vi "GetClampResultNames.vi"(7 "ProjectName":string="Prj", 10 "data":T2={"Clamp Settings"={"Contrast"=40, "Filter width"=4, "Steepness"=2, "Subsampling Ratio"=5, "Show Search Area"=TRUE, "Show Search Lines"=TRUE, "Show Edges Found"=TRUE, "Show Result"=TRUE}, "ROI Descriptor"={"Global Rectangle"=[], "Contours"=[]}, "Process"=0}, 11 "ROI_Name":string="ROI1") -> (3 "ResultNames":string[](array[string]))   [LabVIEW 2019]
uses:
  Controls/Clamp/Analysis_Clamp_Parameter.ctl
  Controls/Clamp/Analysis_Clamp_Result.ctl
panel:
  in  "Analysis_Clamp_Result":T1 {"Edge Point"."Y" format="%.2f"; "Edge Point"."X" format="%.2f"}
  out "error out":errorcluster
  in  "error in (no error)":errorcluster
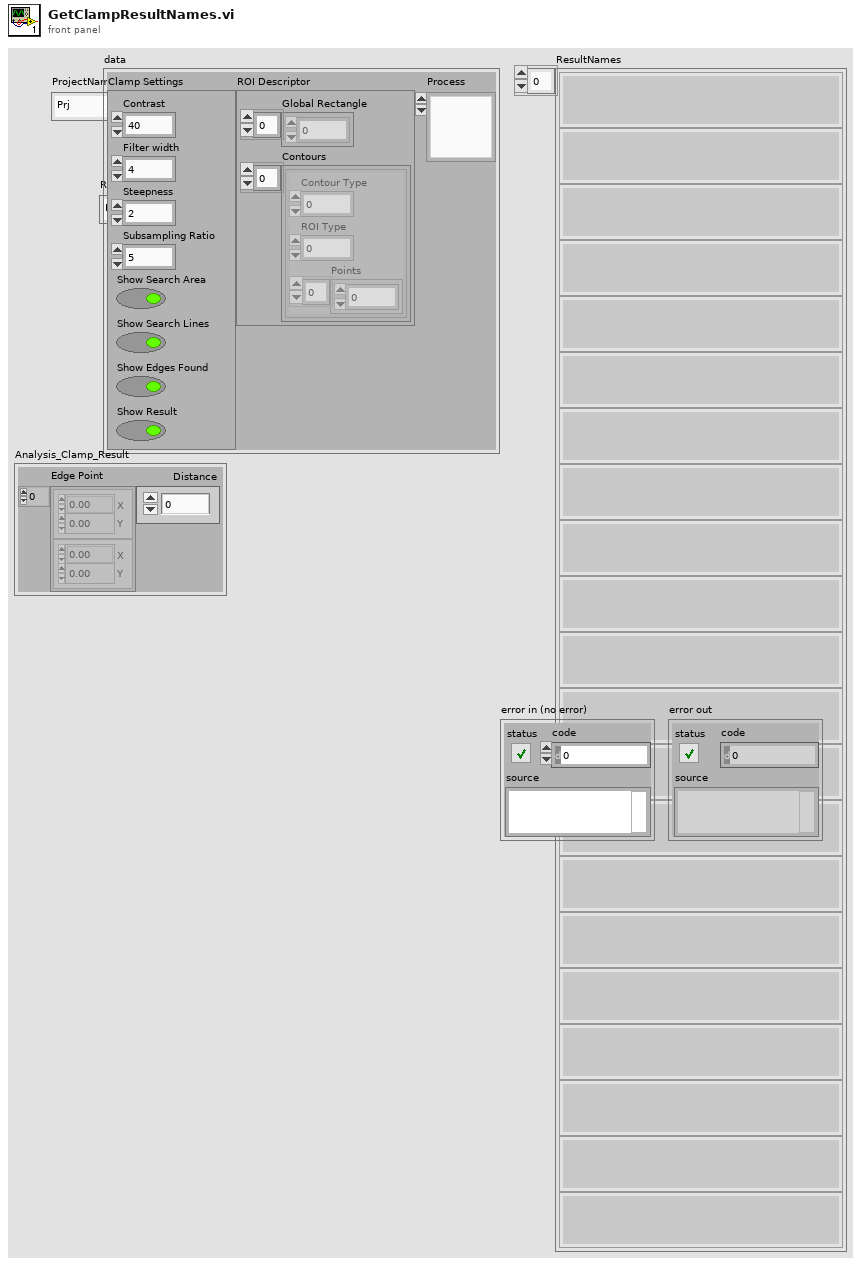
[diagram p1: front panel]
types:
  T1 = typedef "Analysis_Clamp_Result.ctl" = cluster{"Edge Point":cluster{"X":sgl, "Y":sgl}[], "Distance":sgl}
  T2 = typedef "Analysis_Clamp_Parameter.ctl" = cluster{"Clamp Settings":cluster{"Contrast":i32, "Filter width":i32, "Steepness":i32, "Subsampling Ratio":u32, "Show Search Area":bool, "Show Search Lines":bool, "Show Edges Found":bool, "Show Result":bool}, "ROI Descriptor":cluster{"Global Rectangle":i32[], "Contours":cluster{"Contour Type":u32, "ROI Type":u32, "Points":i32[]}[]}, "Process":u16}
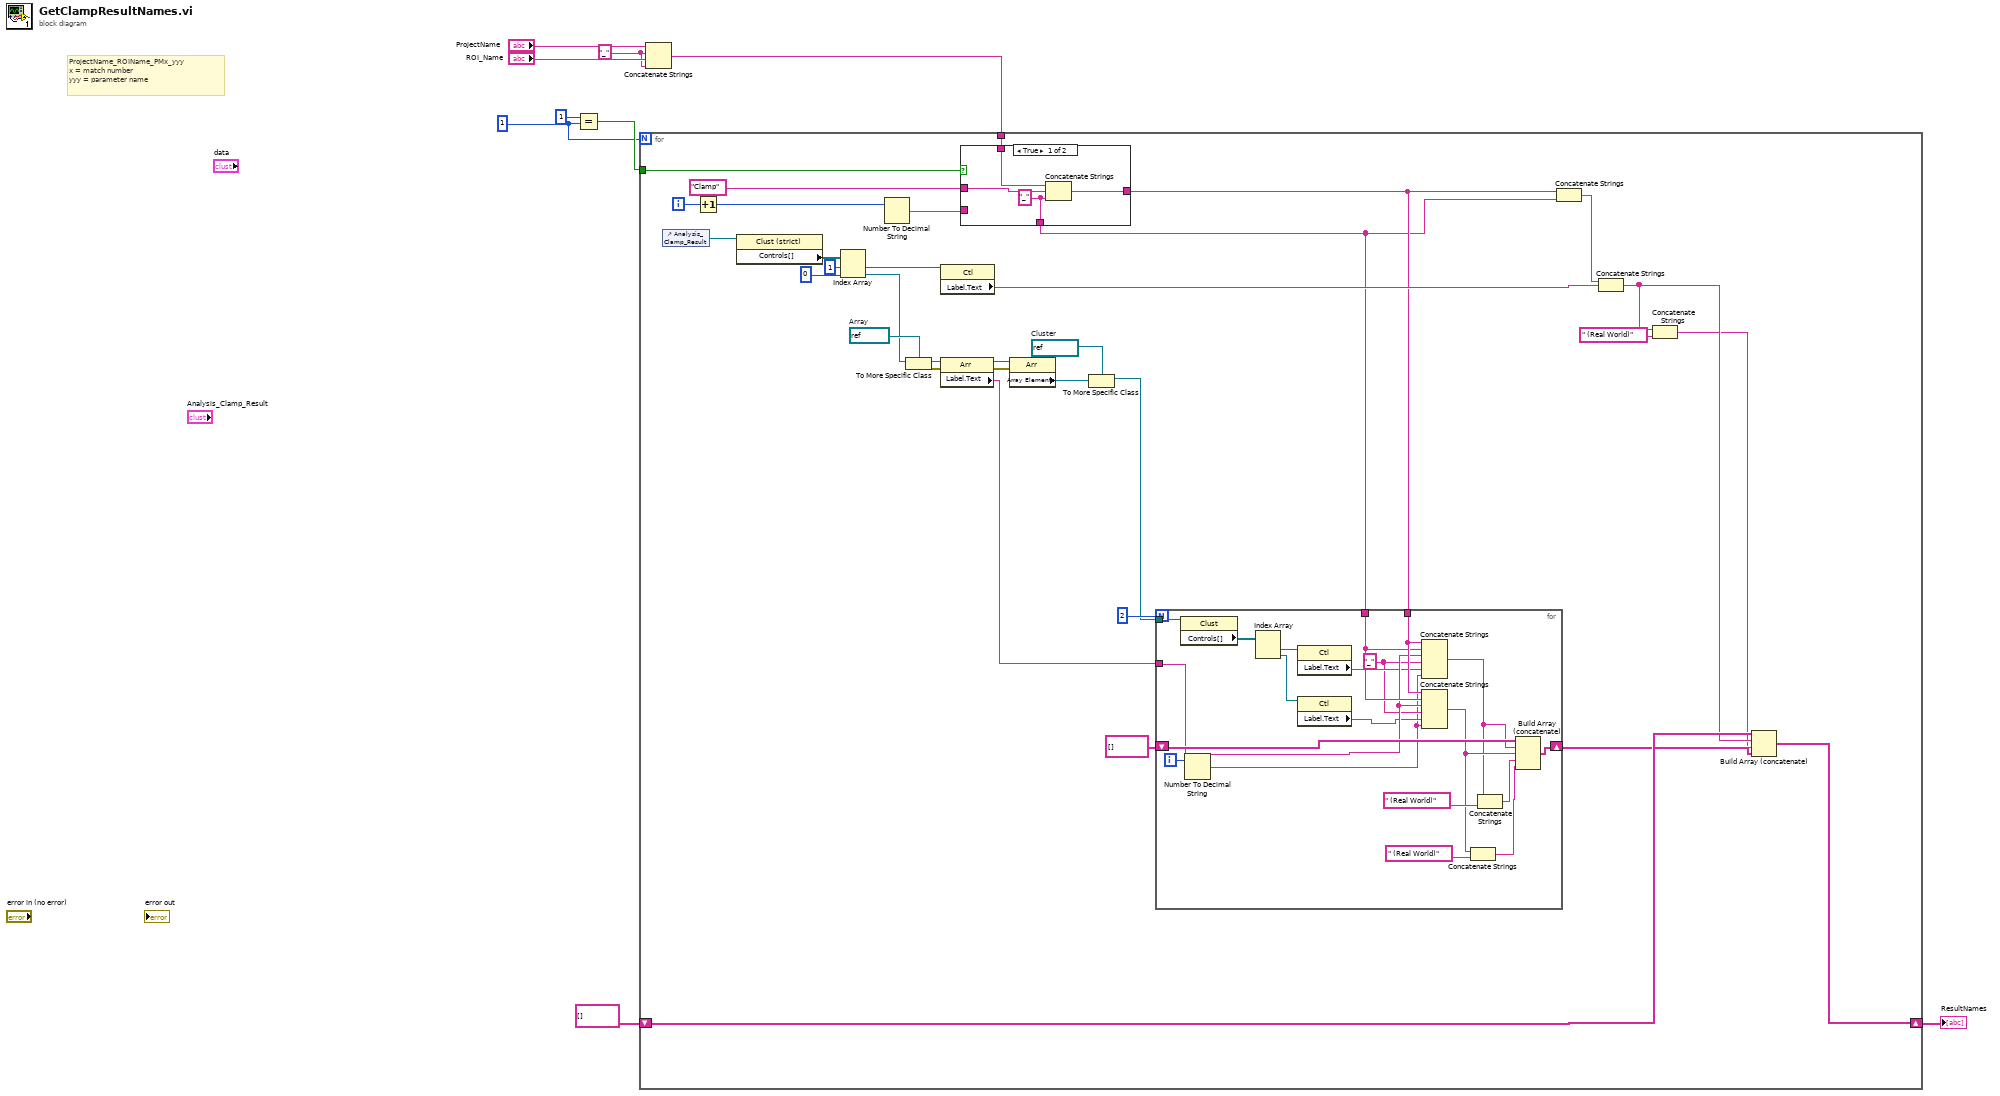
[diagram p0: block diagram]
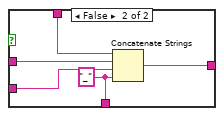
[diagram p2: hidden frame]
diagram:
  w1 = 1
  w6 = "_" ("string")
  # "ProjectName_ROIName_PMx_yyy\nx = match number\nyyy = parameter name"
  n1 = Equal?(x=1, y=w1) -> (x = y?=w2:bool)
  n2 = Concatenate Strings("ProjectName", w6, "ROI_Name", w6) -> (w5:string)
  n3 = for {
    N: w1 -> [_]
    tunnel: w5 -> [w40]
    shift-right: [w32] -> w3
    shift-left: string[] [] -> [w36]
    tunnel: w2 -> [w41]
    i -> [w37]
    w17 = refnum<vi> refnum  # Cluster
    w29 = refnum<vi> refnum  # Array
    n4 = control-ref of="Analysis_Clamp_Result"() -> (w30:refnum<vi>)
    n5 = Increment(x=w37) -> (x+1=w42:i32)
    n6 = property class="Clust (strict)"(reference=w30) -> ("Controls[]"=w34:refnum<vi>[])  [unwired: 1 in, 2 out]
    n7 = Index Array(array=w34, index #1=1 ("index"), index #2=0) -> (element #1=w23:refnum<vi>, element #2=w28:refnum<vi>)
    n8 = Number To Decimal String(number=w42) -> (decimal integer string=w39:string)  [unwired: 1 in]
    n9 = To More Specific Class(target class=w29, reference=w28) -> (specific class reference=w27:refnum<vi>, error out=w26:errorcluster)  [unwired: 1 in]
    n10 = property class="Arr"(reference=w27, error in=w26) -> (reference out=w25:refnum<vi>, error out=w24:errorcluster, "Label.Text"=w14:string)
    n11 = property class="Ctl"(reference=w23) -> ("Label.Text"=w22:string)  [unwired: 1 in, 2 out]
    n12 = case shown="True" w41 {
      tunnel: w40 -> [w66 w71]
      tunnel: w39 -> [_ w69]
      tunnel: [w65 w70] -> w20
      tunnel: "Clamp" ("string") -> [w64 w68]
      tunnel: [w63 w67] -> w19
      frame True {
        w63 = "_" ("string")
        n13 = Concatenate Strings(w66, w64, w63) -> (w65:string)
      }
      frame False {
        w67 = "_" ("string")
        n14 = Concatenate Strings(w71, w68, w69, w67) -> (w70:string)
      }
    }
    n15 = property class="Arr"(reference=w25, error in=w24) -> ("Array Element"=w18:refnum<vi>)  [unwired: 2 out]
    n16 = To More Specific Class(target class=w17, reference=w18) -> (specific class reference=w16:refnum<vi>)  [unwired: 1 in, 1 out]
    n17 = for {
      N: 2 -> [_]
      tunnel: w14 -> [w53]
      tunnel: w16 -> [w62]
      tunnel: w20 -> [w61]
      tunnel: w19 -> [w60]
      shift-right: [w58] -> w11
      shift-left: string[] [] -> [w59]
      i -> [w57]
      w50 = "_" ("string")
      n18 = property class="Clust"(reference=w62) -> ("Controls[]"=w56:refnum<vi>[])  [unwired: 1 in, 2 out]
      n19 = Number To Decimal String(number=w57) -> (decimal integer string=w49:string)  [unwired: 1 in]
      n20 = Index Array(array=w56) -> (element #1=w55:refnum<vi>, element #2=w54:refnum<vi>)  [unwired: 2 in]
      n21 = property class="Ctl"(reference=w55) -> ("Label.Text"=w52:string)  [unwired: 1 in, 2 out]
      n22 = property class="Ctl"(reference=w54) -> ("Label.Text"=w51:string)  [unwired: 1 in, 2 out]
      n23 = Concatenate Strings(w61, w60, w53, w50, w52, w49) -> (w45:string)
      n24 = Concatenate Strings(w61, w60, w53, w50, w51, w49) -> (w47:string)
      n25 = Concatenate Strings(w47, " (Real World)" ("string")) -> (w43:string)
      n26 = Concatenate Strings(w45, " (Real World)" ("string")) -> (w44:string)
      n27 = Build Array (concatenate)(w59, w45, w47, w44, w43) -> (w58:string[])
    }
    n28 = Concatenate Strings(w20, w19) -> (w35:string)
    n29 = Concatenate Strings(w35, w22) -> (w13:string)
    n30 = Concatenate Strings(w13, " (Real World)" ("string")) -> (w10:string)
    n31 = Build Array (concatenate)(w36, w13, w10, w11) -> (w32:string[])
  }
  "ResultNames" <- w3
